vi "K2602 printBuffer.vi"(7 "Channel":enum32{"Channel A", "Channel B"}(ring), 8 "error in (no error)":errorcluster, 9 "End Index":u32, 10 "Start Index":u32, 11 "SMU":refnum<visa-resource-name>="GPIB0::26::INSTR") -> (0 "error out":errorcluster, 1 "V array":dbl[](array[numeric]), 2 "I array":dbl[](array[numeric]), 3 "SMU out":refnum<visa-resource-name>, 4 "End Index out":u32)   [LabVIEW 2012]
uses:
  <instrlib>/KE26XX/KE26XX.lvlib
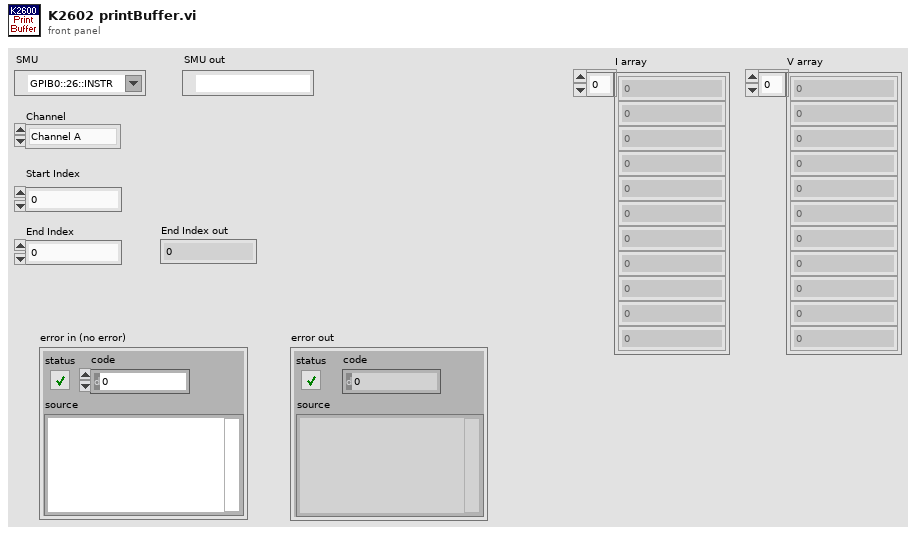
[diagram p1: front panel]
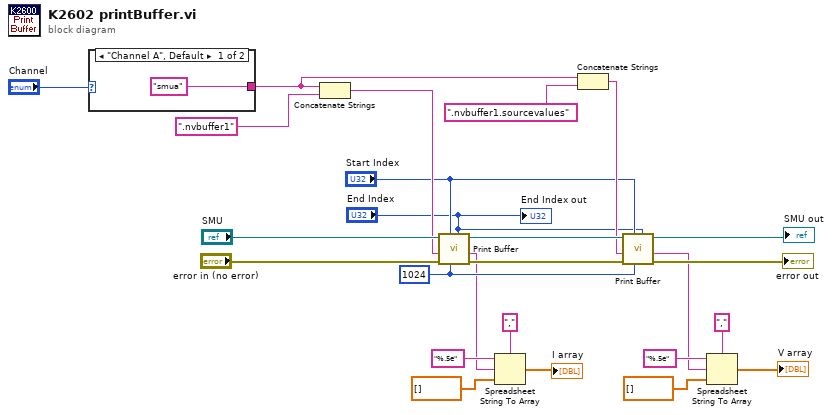
[diagram p0: block diagram]
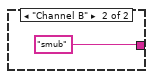
[diagram p2: hidden frame]
diagram:
  w21 = u32 1024 ("Byte Count (1024)")
  n1 = case shown="\"Channel A\", Default" "Channel" {
    tunnel: ["smua" "smub"] -> w15
    frame "Channel A", Default {
    }
    frame "Channel B" {
    }
  }
  n2 = Concatenate Strings(w15, ".nvbuffer1" ("string")) -> (w16:string)
  n3 = call <instrlib>:"Print Buffer.vi"("End Index (1)"="End Index", "Byte Count (1024)"=w21, "Start Index (1)"="Start Index", "error in (no error)"="error in (no error)", "Buffer Name(s)"=w16, "VISA resource name"="SMU") -> ("error out"=w22:errorcluster, "Buffer Data"=w10:string, "VISA resource name out"=w23:refnum<visa-resource-name>)  [unwired: 1 in, 2 out]
  n4 = Spreadsheet String To Array(delimiter (Tab)=",", format string="%.5e", spreadsheet string=w10, array type (2D Dbl)=dbl[] []) -> (array=→"I array":dbl[])
  n5 = Concatenate Strings(w15, ".nvbuffer1.sourcevalues" ("string")) -> (w13:string)
  n6 = call <instrlib>:"Print Buffer.vi"("End Index (1)"="End Index", "Byte Count (1024)"=w21, "Start Index (1)"="Start Index", "error in (no error)"=w22, "Buffer Name(s)"=w13, "VISA resource name"=w23) -> ("error out"=→"error out":errorcluster, "Buffer Data"=w4:string, "VISA resource name out"=→"SMU out":refnum<visa-resource-name>)  [unwired: 1 in, 2 out]
  n7 = Spreadsheet String To Array(delimiter (Tab)=",", format string="%.5e", spreadsheet string=w4, array type (2D Dbl)=dbl[] []) -> (array=→"V array":dbl[])
  "End Index out" <- "End Index"
